vi "openOrCreateAIniCfg.vi"(8 "error in":errorcluster, 10 "prompt":string, 11 "default name":string) -> (0 "error out":errorcluster, 2 "exists":bool, 3 "ini refnum out":refnum<file>)   [LabVIEW 2010]
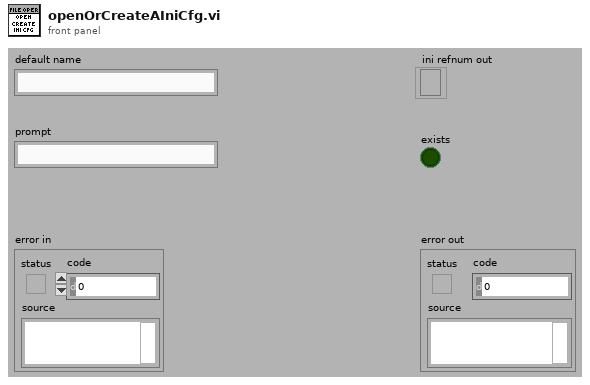
[diagram p1: front panel]
types:
  T1 = enum16{"open", "replace", "create", "open or create", "replace or create", "replace or create with confirmation"}
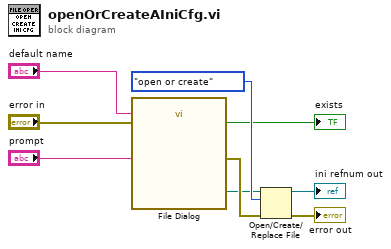
[diagram p0: block diagram]
diagram:
  n1 = call "File Dialog"("prompt"="prompt", "default name"="default name", "error in"="error in") -> ("selected path"=w7:path, "exists"=→"exists":bool, "error out"=w8:errorcluster)  [unwired: 9 in, 1 out]
  n2 = Open/Create/Replace File(file path (use dialog)=w7, error in=w8, operation (0:open)=T1."open or create") -> (refnum out=→"ini refnum out":refnum<file>, error out=→"error out":errorcluster)  [unwired: 3 in, 1 out]
